vi "Keithley DMM7510 Acquire Multipoint.vi"(0 "VISA resource name":refnum<visa-resource-name>="USB0::0x05E6::0x7510::04441973::INSTR", 1 "ID Query (True)":bool=TRUE, 2 "Reset (True)":bool=TRUE, 3 "Auto Range (T: Enable)":bool=TRUE, 5 "error in (no error)":errorcluster, 6 "Tab Control":enum32{"Config", "Measure"}(tab), 7 "Sample Count (10)":i32=10 format="%#.6g", 8 "NPLC":T2=1 items=["0.00005", "0.5", "1", "2", "5", "10", "12", "15"], 9 "Timeout (10000 ms)":i32=20000 format="%#.6g", 10 "Function":T1(ring), 11 "Filter Type":u16(ring) items=["Repeating", "Moving"], 12 "Manual Range (1)":dbl=1e-05, 13 "Enable Filter  (T: Enable)":bool=TRUE) -> (14 "VISA resource name out":refnum<visa-resource-name>, 15 "Measurements":dbl[](array[numeric]) format="%#_9g", 16 "Waveform Chart":dbl[](graph), 17 "Mean":dbl, 19 "error out":errorcluster)   [LabVIEW 2016]
doc: "This example shows how to configure a measurement, set up triggering, trigger a measurement, and retrieve a measurement. It shows how to use the low-level Data VIs to retrieve data from the DMM."
uses:
  <userlib>/_TI-LA/Instr Drivers/Multimeter/Keithley DMM7510/Private/NPLC_Enum.ctl
  <userlib>/_TI-LA/Instr Drivers/Multimeter/Keithley DMM7510/Keithley DMM7510.lvlib
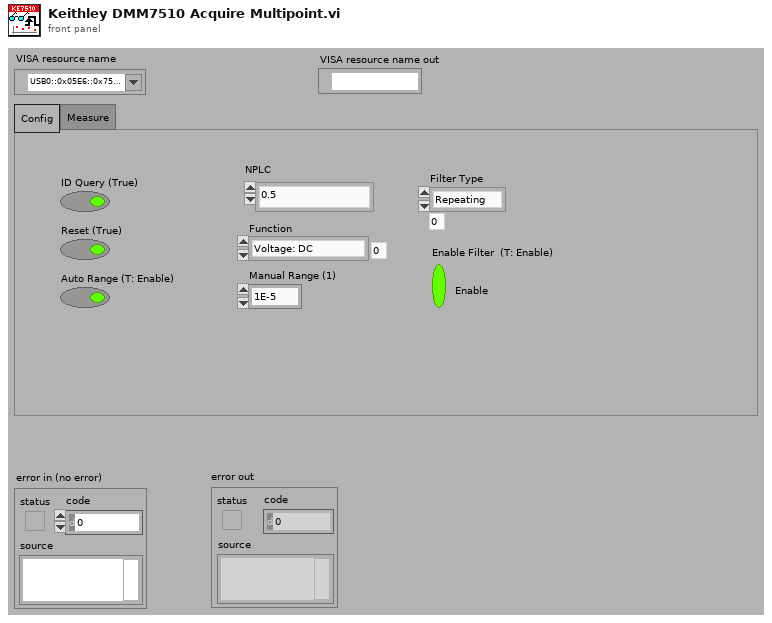
[diagram p1: front panel]
types:
  T1 = enum16{"Voltage: DC", "Voltage: AC", "Current: DC", "Current: AC", "2W Resistance", "4W Resistance", "Diode", "Capacitance", "Temperature", "Continuity", "Frequency", "Period", "Ratio"}
  T2 = typedef "NPLC_Enum.ctl" = u16
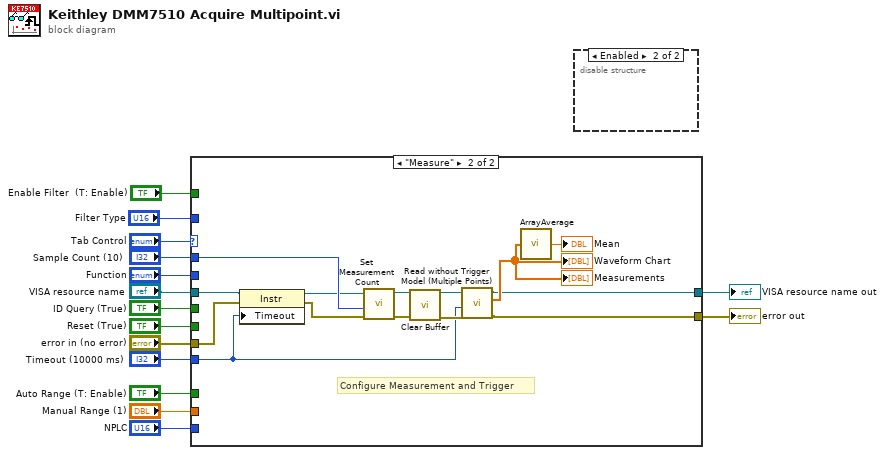
[diagram p0: block diagram]
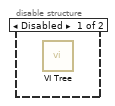
[diagram p2: hidden frame]
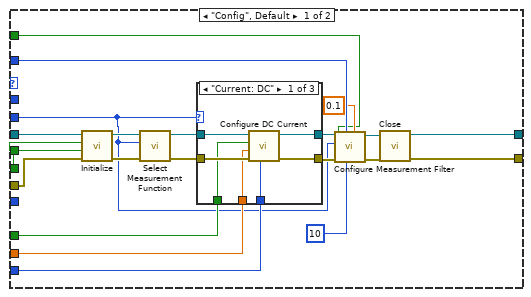
[diagram p3: hidden frame]
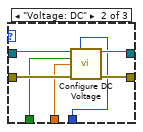
[diagram p4: hidden frame]
diagram:
  n1 = case shown="\"Measure\"" "Tab Control" {
    tunnel: "VISA resource name" -> [w34 w58]
    tunnel: "Function" -> [w17 _]
    tunnel: "Sample Count (10)" -> [_ w66]
    tunnel: "Timeout (10000 ms)" -> [_ w59]
    tunnel: "error in (no error)" -> [w33 w56]
    tunnel: "ID Query (True)" -> [w32 _]
    tunnel: "Reset (True)" -> [w31 _]
    tunnel: [w28 w53] -> w8
    tunnel: [w21 w54] -> w7
    tunnel: "Auto Range (T: Enable)" -> [w27 _]
    tunnel: "Manual Range (1)" -> [w26 _]
    tunnel: "NPLC" -> [w25 _]
    tunnel: "Filter Type" -> [w20 _]
    tunnel: "Enable Filter  (T: Enable)" -> [w18 _]
    frame "Config", Default {
      n2 = call <userlib>:"Initialize.vi"("error in (no error)"=w33, "Reset (True)"=w31, "ID Query (True)"=w32, "VISA resource name"=w34) -> ("error out"=w36:errorcluster, "VISA resource name out"=w35:refnum<visa-resource-name>)  [unwired: 6 in]
      n3 = call <userlib>:"Select Measurement Function.vi"("error in (no error)"=w36, "Function"=w17, "VISA resource name"=w35) -> ("error out"=w29:errorcluster, "VISA resource name out"=w30:refnum<visa-resource-name>)  [unwired: 7 in]
      n4 = case shown="\"Current: DC\"" w17 {
        tunnel: w30 -> [w43 w50 w52]
        tunnel: [w42 w47 w52] -> w24
        tunnel: w29 -> [w40 w49 w51]
        tunnel: [w41 w48 w51] -> w23
        tunnel: w27 -> [w39 w46 _]
        tunnel: w26 -> [w38 w45 _]
        tunnel: w25 -> [w37 w44 _]
        frame "Current: DC" {
          n5 = call <userlib>:"Configure DC Current.vi"("NPLC"=w37, "error in (no error)"=w40, "Manual Range"=w38, "Auto Range? (T: Auto)"=w39, "VISA resource name"=w43) -> ("error out"=w41:errorcluster, "VISA resource name out"=w42:refnum<visa-resource-name>)  [unwired: 5 in]
        }
        frame "Voltage: DC" {
          n6 = call <userlib>:"Configure DC Voltage.vi"("VISA resource name"=w50, "NPLC"=w44, "Auto Range? (T: Auto)"=w46, "Manual Range"=w45, "error in (no error)"=w49) -> ("VISA resource name out"=w47:refnum<visa-resource-name>, "error out"=w48:errorcluster)  [unwired: 9 in]
        }
        frame Default {
        }
      }
      n7 = call <userlib>:"Configure Measurement Filter.vi"("Window"=0.1, "Number of Filter Readings (10)"=u32 10, "Filter Type"=w20, "error in (no error)"=w23, "Enable Filter  (T: Enable)"=w18, "Function"=w17, "VISA resource name"=w24) -> ("error out"=w22:errorcluster, "VISA resource name out"=w21:refnum<visa-resource-name>)  [unwired: 3 in]
      n8 = call <userlib>:"Close.vi"("error in (no error)"=w22, "VISA resource name"=w21) -> ("error out"=w28:errorcluster)  [unwired: 9 in]
    }
    frame "Measure" {
      # "Configure Measurement and Trigger"
      n9 = property class="Instr"(reference=w58, error in=w56, "Timeout"=w59) -> (reference out=w57:refnum<visa-resource-name>, error out=w55:errorcluster)
      n10 = call <userlib>:"Set Measurement Count.vi"("error in (no error)"=w55, "Count"=w66, "VISA resource name"=w57) -> ("error out"=w65:errorcluster, "VISA resource name out"=w64:refnum<visa-resource-name>)  [unwired: 7 in]
      n11 = call <userlib>:"Clear Buffer.vi"("VISA resource name"=w64, "error in (no error)"=w65) -> ("VISA resource name out"=w63:refnum<visa-resource-name>, "error out"=w62:errorcluster)  [unwired: 12 in]
      n12 = call <userlib>:"Read without Trigger Model (Multiple Points).vi"("error in (no error)"=w62, "Timeout (10000 ms)"=w59, "VISA resource name"=w63) -> ("error out"=w53:errorcluster, "Measurements"=w60:dbl[], "VISA resource name out"=w54:refnum<visa-resource-name>)  [unwired: 5 in, 1 out]
      "Waveform Chart" <- w60
      "Measurements" <- w60
      n13 = call "ArrayAverage.vi"("InputArray"=w60) -> ("AvgOut"=→"Mean":dbl)  [unwired: 4 in]
    }
  }
  "error out" <- w8
  "VISA resource name out" <- w7
  n14 = disable-structure shown="Enabled" {
    frame Disabled {
      n15 = call <userlib>:"VI Tree.vi"() -> ()  [unwired: 12 in]
    }
    frame Enabled {
    }
  }
